vi "loadRangeInUse.vi"(6 "type":string, 8 "error in (no error)":errorcluster, 9 "device.lvclass":refnum<class "device.lvclass">, 10 "NativeXML in":refnum<class "NativeXML.lvclass">, 11 "deviceDataBase in":refnum<class "deviceDataBase.lvclass">) -> (0 "error out":errorcluster, 1 "device.lvclass out":refnum<class "device.lvclass">, 2 "NativeXML out":refnum<class "NativeXML.lvclass">, 3 "deviceDataBase out":refnum<class "deviceDataBase.lvclass">)   [LabVIEW 2011, in "Tools.lvlib" / "DatabaseHelpers.lvlib" / "deviceDataBase.lvclass"]
uses:
  deviceDataBase.lvclass
  NativeXML/NativeXML.lvclass
  Database Objects/device/device.lvclass
  Database Objects/device/AnalogDevice/AnalogDevice.lvclass
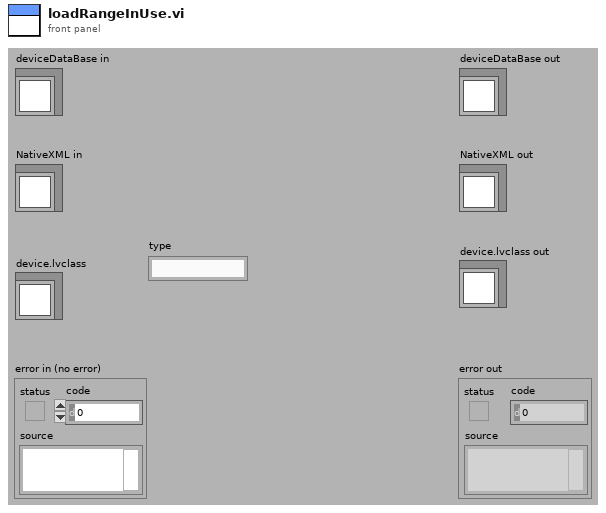
[diagram p1: front panel]
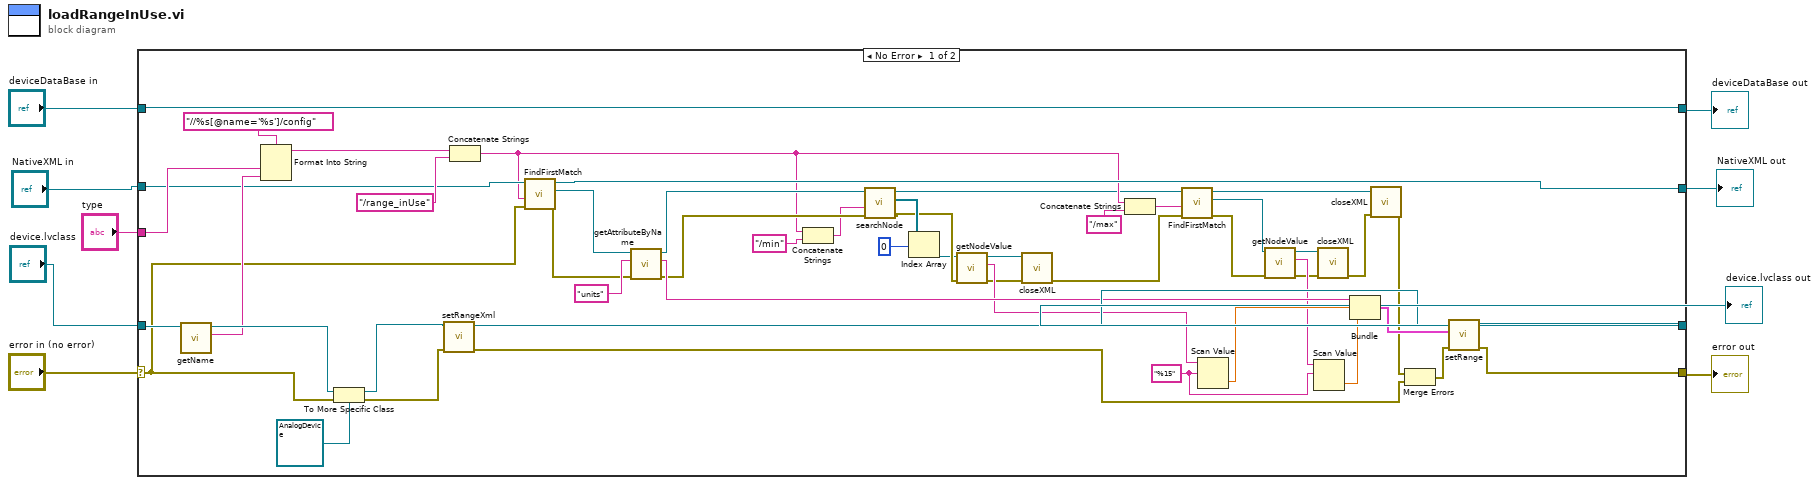
[diagram p0: block diagram]
diagram:
  n1 = case shown="No Error" "error in (no error)" {
    selector: "error in (no error)" -> [w22 w62]
    tunnel: [w38 w62] -> w2
    tunnel: [w60 w61] -> w5
    tunnel: "deviceDataBase in" -> [w60 w61]
    tunnel: "NativeXML in" -> [w23 _]
    tunnel: "device.lvclass" -> [w31 _]
    tunnel: [w58 _] -> w3
    tunnel: [w24 _] -> w4
    tunnel: "type" -> [w28 _]
    frame No Error {
      w56 = "%15"
      n2 = call "getName.vi"("device.lvclass in"=w31) -> ("name"=w27:string, "device.lvclass out"=w30:refnum<class "device.lvclass">)  [unwired: 8 in, 1 out]
      n3 = Format Into String(format string="//%s[@name='%s']/config", w28, w27) -> (resulting string=w26:string)  [unwired: 2 in, 1 out]
      n4 = To More Specific Class(target class=refnum<class "AnalogDevice.lvclass"> refnum ("Tools.lvlib:DatabaseHelpers.lvlib:AnalogDevice.lvclass"), reference=w30, error in=w22) -> (specific class reference=w51:refnum<class "AnalogDevice.lvclass">, error out=w49:errorcluster)
      n5 = call "setRangeXml.vi"("error in (no error)"=w49, "AnalogDevice in"=w51) -> ("error out"=w48:errorcluster, "AnalogDevice out"=w50:refnum<class "AnalogDevice.lvclass">)  [unwired: 8 in]
      n6 = Concatenate Strings(w26, "/range_inUse") -> (w16:string)
      n7 = call "FindFirstMatch.vi"("error in (no error)"=w22, "xPath"=w16, "NativeXML in"=w23) -> ("error out"=w21:errorcluster, "NativeXML match"=w20:refnum<class "NativeXML.lvclass">, "NativeXML out"=w24:refnum<class "NativeXML.lvclass">)  [unwired: 6 in]
      n8 = call "getAttributeByName.vi"("error in (no error)"=w21, "name"="units", "NativeXML in"=w20) -> ("error out"=w45:errorcluster, "Attribute String"=w46:string, "NativeXML out"=w43:refnum<class "NativeXML.lvclass">)  [unwired: 6 in]
      n9 = Concatenate Strings(w16, "/min") -> (w18:string)
      n10 = call "searchNode.vi"("error in (no error)"=w45, "searchXPath"=w18, "NativeXML in"=w43) -> ("error out"=w42:errorcluster, "nodeArray"=w44:refnum<class "NativeXML.lvclass">[], "NativeXML out"=w15:refnum<class "NativeXML.lvclass">)  [unwired: 6 in]
      n11 = Index Array(array=w44, index=0) -> (element=w41:refnum<class "NativeXML.lvclass">)
      n12 = call "getNodeValue.vi"("error in (no error)"=w42, "NativeXML in"=w41) -> ("error out"=w34:errorcluster, "Value"=w40:string, "NativeXML out"=w35:refnum<class "NativeXML.lvclass">)  [unwired: 7 in]
      n13 = call "closeXML.vi"("error in (no error)"=w34, "NativeXML in"=w35) -> ("error out"=w13:errorcluster)  [unwired: 9 in]
      n14 = Concatenate Strings(w16, "/max") -> (w14:string)
      n15 = call "FindFirstMatch.vi"("error in (no error)"=w13, "xPath"=w14, "NativeXML in"=w15) -> ("error out"=w12:errorcluster, "NativeXML match"=w11:refnum<class "NativeXML.lvclass">, "NativeXML out"=w10:refnum<class "NativeXML.lvclass">)  [unwired: 6 in]
      n16 = Scan Value(string=w40, format string=w56) -> (value=w57:dbl)  [unwired: 1 in, 1 out]
      n17 = call "getNodeValue.vi"("error in (no error)"=w12, "NativeXML in"=w11) -> ("error out"=w37:errorcluster, "Value"=w39:string, "NativeXML out"=w36:refnum<class "NativeXML.lvclass">)  [unwired: 7 in]
      n18 = Scan Value(string=w39, format string=w56) -> (value=w55:dbl)  [unwired: 1 in, 1 out]
      n19 = call "closeXML.vi"("error in (no error)"=w37, "NativeXML in"=w36) -> ("error out"=w33:errorcluster)  [unwired: 9 in]
      n20 = Bundle("Attribute String"=w46, w57, w55) -> (w54:cluster{"Attribute String":string, dbl, dbl})  [unwired: 1 in]
      n21 = call "closeXML.vi"("error in (no error)"=w33, "NativeXML in"=w10) -> ("error out"=w32:errorcluster)  [unwired: 9 in]
      n22 = Merge Errors(w32, w48) -> (w53:errorcluster)
      n23 = call "setRange.vi"("error in (no error)"=w53, "Range"=w54, "AnalogDevice.lvclass in"=w50) -> ("error out"=w38:errorcluster, "AnalogDevice.lvclass out"=w58:refnum<class "AnalogDevice.lvclass">)  [unwired: 7 in]
    }
    frame Error {
    }
  }
  "error out" <- w2
  "deviceDataBase out" <- w5
  "device.lvclass out" <- w3
  "NativeXML out" <- w4
